vi "Swap Slot.vi"(8 "error in":errorcluster, 10 "slot 2 ref in":T1 format="%.0x", 11 "slot 1 ref in":T1 format="%.0x") -> (0 "error out":errorcluster, 2 "slot 2 ref out":T1 format="%.0x", 3 "slot 1 ref out":T1 format="%.0x")   [LabVIEW 2017, in "Scan Engine Scripting.lvlib"]
uses:
  Scan Engine Scripting.lvlib
  <vilib>/NI Veristand/Custom Device API/Custom Device Item Ref.ctl
  Modules.lvlibp/RSI Module/RSI Module.lvclass
  Scan Engine Custom Device.lvlib
  <vilib>/NI Veristand/Custom Device API/Custom Device API.lvlib
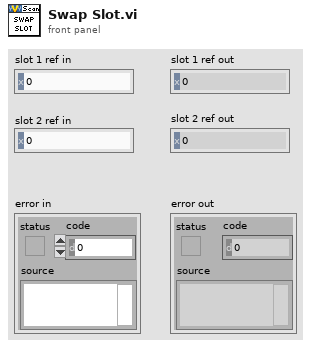
[diagram p1: front panel]
types:
  T1 = typedef "Custom Device API.lvlib/Custom Device Item Ref.ctl" = u64
  T2 = typedef "Modules.lvlibp/Custom Device API.lvlib/Custom Device Item Ref.ctl" = u64
  T3 = cluster{"Node Ptr Out":T2, "RSI Module out":refnum<class "RSI Module.lvclass">}
  T4 = cluster{"Node Ptr Out":T2, "RSI Module out":refnum<class "RSI Module.lvclass">}[]
  T5 = typedef "Modules.lvlibp/RSI Module.lvclass/Module Models.ctl" = enum16{"Empty", "NI 9201", "NI 9203", "NI 9205", "NI 9206", "NI 9207", "NI 9208", "NI 9209", "NI 9210", "NI 9211", "NI 9212", "NI 9213", "NI 9214", "NI 9215", "NI 9216", "NI 9217", "NI 9219", "NI 9220", "NI 9221", "NI 9222", "NI 9223", "NI 9224", "NI 9225", "NI 9226", "NI 9227", "NI 9228", "NI 9229", "NI 9233", "NI 9234", "NI 9235", "NI 9236", "NI 9237", "NI 9239", "NI 9242", "NI 9244", "NI 9253", "NI 9263", "NI 9264", "NI 9265", "NI 9266", "NI 9269", "NI 9344", "NI 9350", "NI 9375", "NI 9401", "NI 9402", "NI 9403", "NI 9411", "NI 9421", "NI 9422", "NI 9423", "NI 9425", "NI 9426", "NI 9435", "NI 9436", "NI 9437", "NI 9472", "NI 9474", "NI 9475", "NI 9476", "NI 9477", "NI 9478", "NI 9481", "NI 9482", "NI 9485"}
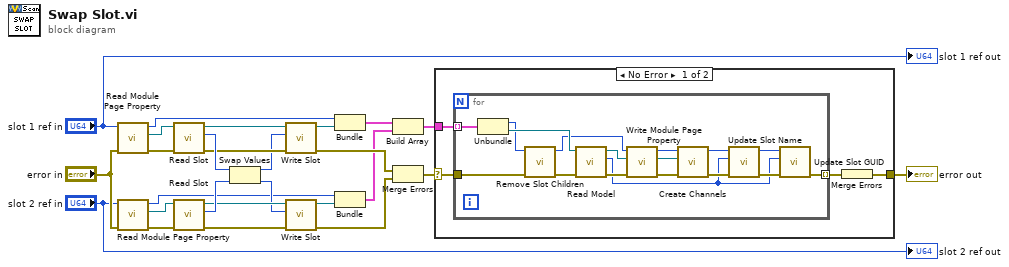
[diagram p0: block diagram]
diagram:
  n1 = call "Read Module Page Property.vi"("error in (no error)"="error in", "Node Ptr In"="slot 1 ref in") -> ("error out"=w26:errorcluster, "RSI Module"=w25:refnum<class "RSI Module.lvclass">, "Node Ptr Out"=w10:T2)  [unwired: 7 in]
  n2 = call "Read Module Page Property.vi"("error in (no error)"="error in", "Node Ptr In"="slot 2 ref in") -> ("error out"=w23:errorcluster, "RSI Module"=w24:refnum<class "RSI Module.lvclass">, "Node Ptr Out"=w7:T2)  [unwired: 7 in]
  n3 = call "Read Slot.vi"("error in (no error)"=w26, "RSI Module in"=w25) -> ("error out"=w16:errorcluster, "Slot"=w21:u32, "RSI Module out"=w19:refnum<class "RSI Module.lvclass">)  [unwired: 7 in]
  n4 = call "Read Slot.vi"("error in (no error)"=w23, "RSI Module in"=w24) -> ("error out"=w17:errorcluster, "Slot"=w20:u32, "RSI Module out"=w18:refnum<class "RSI Module.lvclass">)  [unwired: 7 in]
  n5 = Swap Values(12:w21, 14:w20) -> (1:w15:u32, 3:w14:u32)  [unwired: 1 in]
  n6 = call "Write Slot.vi"("error in (no error)"=w16, "Slot"=w15, "RSI Module in"=w19) -> ("error out"=w11:errorcluster, "RSI Module out"=w9:refnum<class "RSI Module.lvclass">)  [unwired: 7 in]
  n7 = call "Write Slot.vi"("error in (no error)"=w17, "Slot"=w14, "RSI Module in"=w18) -> ("error out"=w13:errorcluster, "RSI Module out"=w8:refnum<class "RSI Module.lvclass">)  [unwired: 7 in]
  n8 = Bundle("Node Ptr Out"=w10, "RSI Module out"=w9) -> (w6:T3)  [unwired: 1 in]
  n9 = Bundle("Node Ptr Out"=w7, "RSI Module out"=w8) -> (w5:T3)  [unwired: 1 in]
  n10 = Build Array(w6, w5) -> (w4:T4)
  n11 = Merge Errors(w11, w13) -> (w12:errorcluster)
  n12 = case shown="No Error" w12 {
    selector: w12 -> [w30 w48]
    tunnel: w4 -> [w29 _]
    tunnel: [w27 w48] -> w3
    frame No Error {
      n13 = for {
        tunnel: w30 -> [w34]
        tunnel: w29 -> [w41] mode=indexing
        tunnel: [w35] -> w28 mode=indexing
        n14 = Unbundle(w41) -> ("Node Ptr Out"=w32:T2, "RSI Module out"=w40:refnum<class "RSI Module.lvclass">)
        n15 = call "Remove Slot Children.vi"("error in (no error)"=w34, "slot ref in"=w32) -> ("error out"=w33:errorcluster, "slot ref out"=w31:T1)  [unwired: 8 in]
        n16 = call "Read Model.vi"("error in (no error)"=w33, "RSI Module in"=w40) -> ("error out"=w42:errorcluster, "Model"=w38:T5, "RSI Module out"=w43:refnum<class "RSI Module.lvclass">)  [unwired: 7 in]
        n17 = call "Write Module Page Property.vi"("error in (no error)"=w42, "RSI Module"=w43, "Node Ptr In"=w31) -> ("error out"=w45:errorcluster, "RSI Module out"=w47:refnum<class "RSI Module.lvclass">, "Node Ptr Out"=w39:T2)  [unwired: 6 in]
        n18 = call-dynamic "Create Channels.vi"("error in (no error)"=w45, "RSI Module in"=w47, "Parent Ref in"=w39) -> ("error out"=w46:errorcluster, "Parent Ref out"=w37:T2)  [unwired: 6 in, 1 out]
        n19 = call "Update Slot Name.vi"("error in"=w46, "module"=w38, "slot ref in"=w37) -> ("error out"=w44:errorcluster, "slot ref out"=w36:T1)  [unwired: 6 in, 1 out]
        n20 = call "Update Slot GUID.vi"("error in"=w44, "module model"=w38, "slot ref in"=w36) -> ("error out"=w35:errorcluster)  [unwired: 7 in, 1 out]
      }
      n21 = Merge Errors(w28) -> (w27:errorcluster)
    }
    frame Error {
    }
  }
  "error out" <- w3
  "slot 1 ref out" <- "slot 1 ref in"
  "slot 2 ref out" <- "slot 2 ref in"
